vi "SetupEOM.vi"() -> ()   [LabVIEW 2009]
uses:
  EOMSettings.ctt
panel:
  in  "Analog Setup":bool
  in  "Cancel Button":bool
  in  "OK Button":bool
  in  "EOM Settings":T1={"Output Channel"="1", "EOM Voltage"=10.0, "Pixel per Polymode Cycle"=10, "Time per Polymode Cycle"=5.0} {"Time per Polymode Cycle" format="%.2f"; "Pixel per Polymode Cycle" max=20 step=1; "EOM Voltage" min=0.0 max=20.0 step=0.1 format="%.2f"}
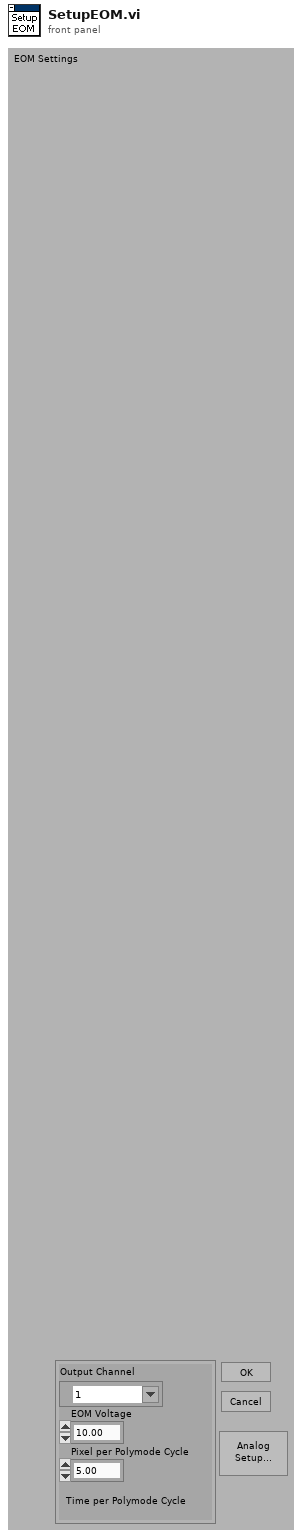
[diagram p1: front panel]
types:
  T1 = typedef "EOMSettings.ctt" = cluster{"Output Channel":tag, "EOM Voltage":dbl, "Pixel per Polymode Cycle":u32, "Time per Polymode Cycle":dbl}
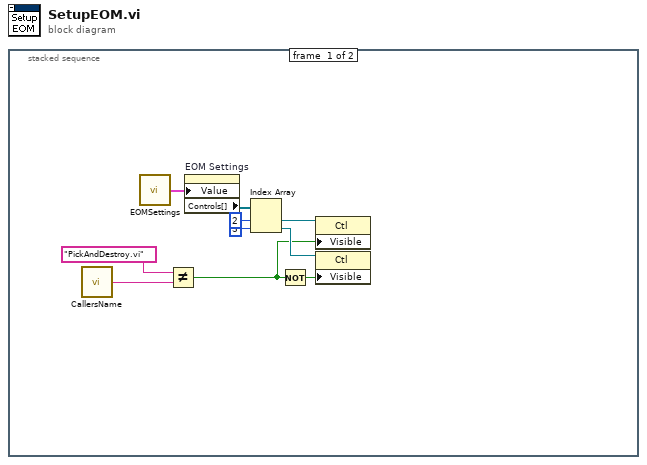
[diagram p0: block diagram]
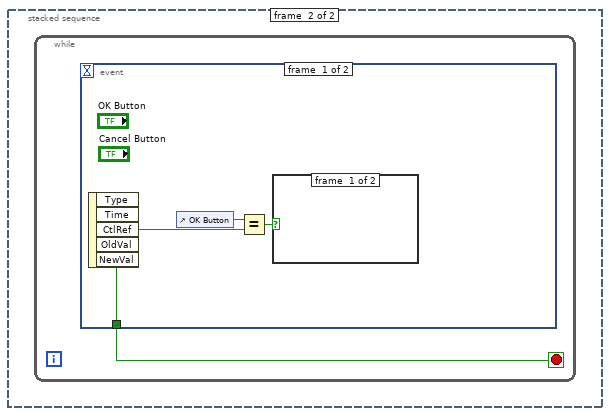
[diagram p2: hidden frame]
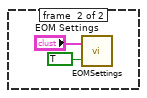
[diagram p3: hidden frame]
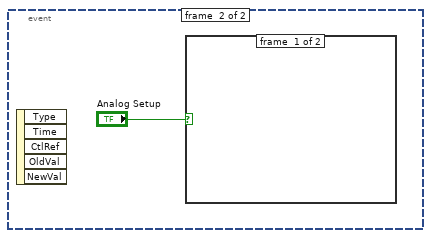
[diagram p4: hidden frame]
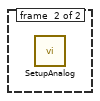
[diagram p5: hidden frame]
diagram:
  n1 = stacked-sequence {
    frame #0 {
      n2 = call "CallersName.vi"() -> ("Callers Name out"=w4:string)  [unwired: 2 in]
      n3 = call "EOMSettings.vi"() -> ("EOM Settings (output)"=w10:T1)  [unwired: 2 in]
      n4 = Not Equal?(x="PickAndDestroy.vi", y=w4) -> (x != y?=w1:bool)
      n5 = property on="EOM Settings" class="Clust (strict)"("Value"=w10) -> ("Controls[]"=w9:refnum<vi>[])  [unwired: 2 in, 2 out]
      n6 = Index Array(array=w9, index #1=2 ("index"), index #2=3 ("index")) -> (element #1=w6:refnum<vi>, element #2=w5:refnum<vi>)
      n7 = Not(x=w1) -> (.not. x?=w2:bool)
      n8 = property class="Ctl"(reference=w6, "Visible"=w1) -> ()  [unwired: 1 in, 2 out]
      n9 = property class="Ctl"(reference=w5, "Visible"=w2) -> ()  [unwired: 1 in, 2 out]
    }
    frame #1 {
      n10 = while {
        stop <- w11 stop-if-true
        n11 = event shown="[1] \"Analog Setup\": Value Change" {
          selector: _ -> [_ _]
          dyn-events: _ -> [_ _]
          timeout: _ -> [_ _]
          tunnel: [w14 _] -> w11
          event #0 {
            n12 = event-data() -> ("CtlRef"=w15:refnum<vi>, "NewVal"=w14:bool)  [unwired: 1 in, 3 out]
            n13 = control-ref of="OK Button"() -> (w13:refnum<vi>)
            n14 = Equal?(x=w13, y=w15) -> (x = y?=w12:bool)
            n15 = case shown="True" w12 {
              frame #0 {
              }
              frame #1 {
                n16 = call "EOMSettings.vi"("Get/Set"=TRUE, "EOM Settings (input)"="EOM Settings") -> ()  [unwired: 1 out]
              }
            }
          }
          event #1 {
            n17 = event-data() -> ()  [unwired: 1 in, 5 out]
            n18 = case shown="True" "Analog Setup" {
              frame #0 {
              }
              frame #1 {
                n19 = call "SetupAnalog.vi"() -> ()  [unwired: 1 in]
              }
            }
          }
        }
      }
    }
  }
